vi "FTW-Linker-LVFileStaticLinks.vi"(8 "error in":errorcluster, 10 "Recursive":bool=TRUE, 11 "LabVIEW Files":path[](array[path])) -> (0 "error out":errorcluster, 3 "LinkerInfo":T1[](array[typedef]) {"iState" format="%08x"; "iStyle" format="%08x"; "wStyle" format="%08x"; "buttons" format="%08x"; "viflags" format="%08x"; "viflags2" format="%08x"})   [LabVIEW 2015]
uses:
  FTW-Linker-LinkerInfoStructure.ctl
  FTW-Linker-LabVIEWFiletype.ctl
panel:
  # "Inputs"
  # "Outputs"
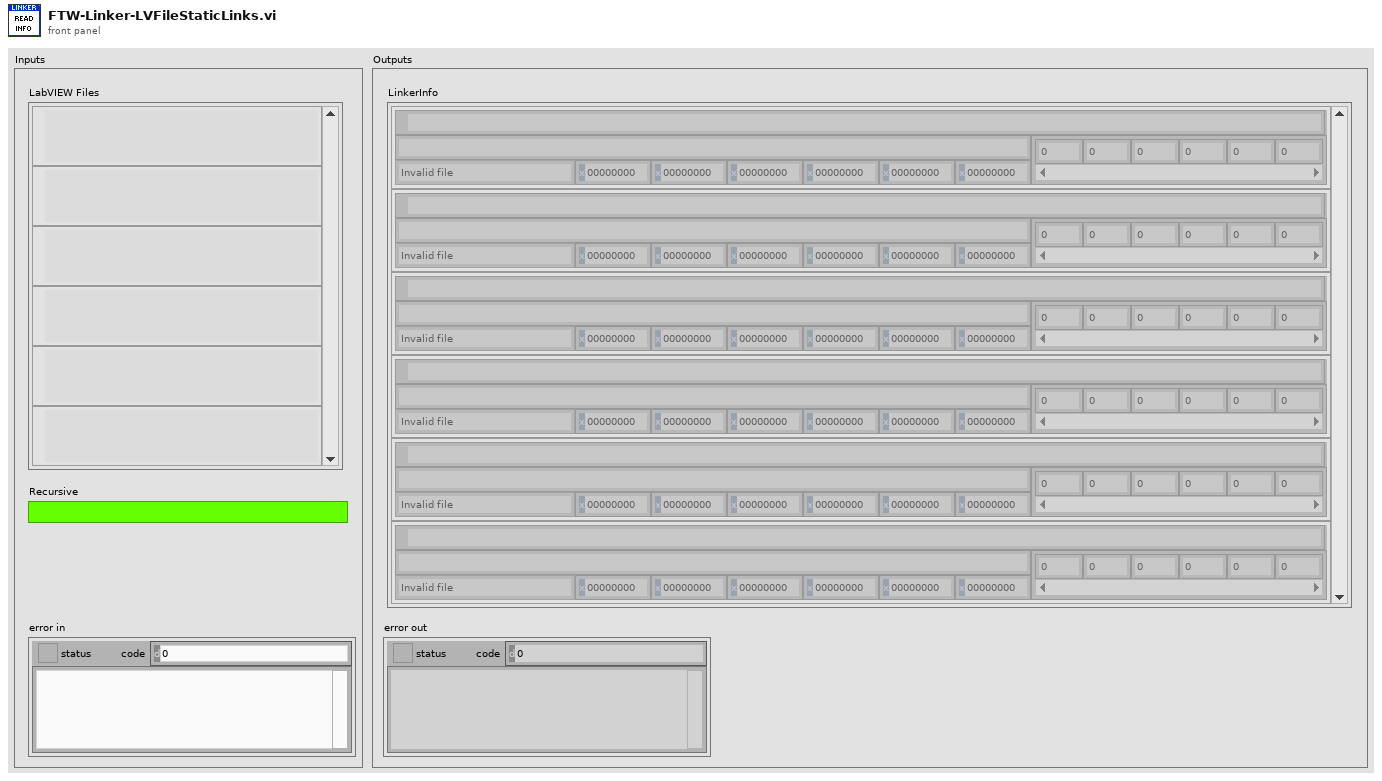
[diagram p1: front panel]
types:
  T1 = typedef "FTW-Linker-LinkerInfoStructure.ctl" = cluster{"path":path, "delimited name":string, "Filetype":T2, "iState":u32, "iStyle":u16, "wStyle":u16, "buttons":u16, "viflags":u32, "viflags2":u32, "links":u32[]}
  T2 = typedef "FTW-Linker-LabVIEWFiletype.ctl" = enum32{"Invalid file", "Unknown type", "Instrument", "Control", "Polymorphic VI", "Project", "Library", "LVClass", "XControl", "XNode", "Shared library", ".NET assembly", "ActiveX interface", "CIN", "Run-time menu", "Palette menu", "Help file", "LLB", "XNode Edit Dependency", "Class Private Data Control", "Statechart", "MathScript .m file", "Ladder Diagram", "LVLibp", "XNode Build Dependency"}
  T3 = typedef "NI_FileType.lvlib/LVFileType.ctl" = enum32{"Invalid file", "Unknown type", "Instrument", "Control", "Polymorphic VI", "Project", "Library", "LVClass", "XControl", "XNode", "Shared library", ".NET assembly", "ActiveX interface", "CIN", "Run-time menu", "Palette menu", "Help file", "LLB", "XNode Edit Dependency", "Class Private Data Control", "Statechart", "MathScript .m file", "Ladder Diagram", "LVLibp", "XNode Build Dependency"}
  T4 = cluster{"path":path, "delimited name":string, "type":T3, "iState":u32, "iStyle":u16, "wStyle":u16, "buttons":u16, "viflags":u32, "viflags2":u32, "links":u32[]}[]
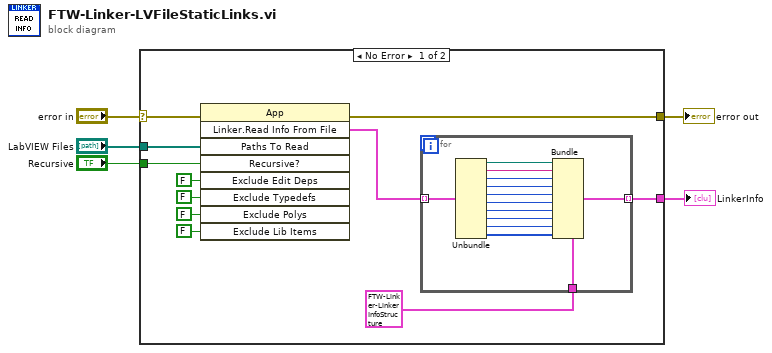
[diagram p0: block diagram]
diagram:
  n1 = case shown="No Error" "error in" {
    selector: "error in" -> [w10 w30]
    tunnel: [w16 w30] -> w5
    tunnel: "Recursive" -> [w15 _]
    tunnel: [w13 _] -> w3
    tunnel: "LabVIEW Files" -> [w11 _]
    frame No Error {
      n2 = invoke class="App" method="Linker.Read Info From File"(error in=w10, "Paths To Read"=w11, "Recursive?"=w15, "Exclude Edit Deps"=FALSE ("Exclude Edit Time Dependencies"), "Exclude Typedefs"=FALSE, "Exclude Polys"=FALSE ("Exclude Poly VIs"), "Exclude Lib Items"=FALSE ("Exclude Unused Library Items")) -> (error out=w16:errorcluster, "Linker.Read Info From File"=w14:T4)  [unwired: 2 in, 7 out]
      n3 = for {
        tunnel: w14 -> [w29] mode=indexing
        tunnel: [w27] -> w13 mode=indexing
        tunnel: T1 {"path"=path "", "delimited name"="", "Filetype"=enum."Invalid file", "iState"=0, "iStyle"=0, "wStyle"=0, "buttons"=0, "viflags"=0, "viflags2"=0, "links"=[]} ("Linker Info") -> [w28]
        n4 = Unbundle(w29) -> ("path"=w26:path, "delimited name"=w25:string, "type"=w17:T3, "iState"=w24:u32, "iStyle"=w23:u16, "wStyle"=w22:u16, "buttons"=w21:u16, "viflags"=w20:u32, "viflags2"=w19:u32, "links"=w18:u32[])
        n5 = Bundle(cluster=w28, "path"=w26, "delimited name"=w25, "Filetype"=w17, "iState"=w24, "iStyle"=w23, "wStyle"=w22, "buttons"=w21, "viflags"=w20, "viflags2"=w19, "links"=w18) -> (w27:T1)
      }
    }
    frame Error {
    }
  }
  "error out" <- w5
  "LinkerInfo" <- w3
